vi "UpdateScrollbar.vi"(6 "# Cols":u32=1, 7 "Value Scrollbar":i32, 8 "error in":errorcluster, 9 "#Rows":u32=7, 10 "# Elements":i32, 11 "Cluster Refnum":refnum<vi>) -> (0 "error out":errorcluster)   [LabVIEW 2020, in "FakedArray.lvclass"]
uses:
  FakedArray.lvclass
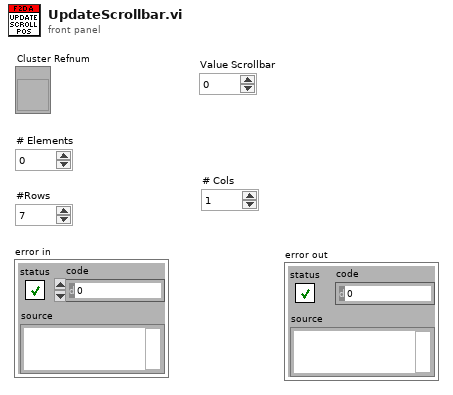
[diagram p1: front panel]
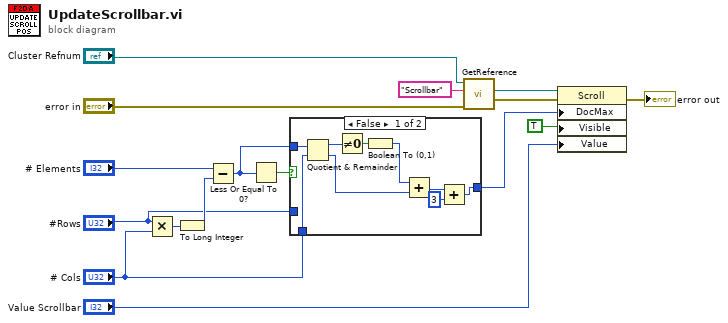
[diagram p0: block diagram]
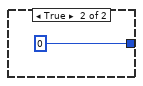
[diagram p2: hidden frame]
diagram:
  n1 = Multiply(x="#Rows", y="# Cols") -> (x*y=w2:u32)
  n2 = To Long Integer(number=w2) -> (32bit integer=w5:i32)
  n3 = Subtract(x="# Elements", y=w5) -> (x-y=w16:i32)
  n4 = Less Or Equal To 0?(x=w16) -> (x <= 0?=w13:bool)
  n5 = case shown="False" w13 {
    tunnel: [w18 0] -> w14
    tunnel: w16 -> [w25 _]
    tunnel: "# Cols" -> [w24 _]
    tunnel: "#Rows" -> [_ _]
    frame False {
      n6 = Quotient & Remainder(x=w25, y=w24) -> (x-y*floor(x/y)=w23:u32, floor(x/y)=w20:u32)
      n7 = Not Equal To 0?(x=w23) -> (x != 0?=w22:bool)
      n8 = Boolean To (0,1)(Boolean=w22) -> (0, 1=w21:i16)
      n9 = Add(x=w21, y=w20) -> (x+y=w19:u32)
      n10 = Add(x=w19, y=u32 3) -> (x+y=w18:u32)
    }
    frame True {
    }
  }
  n11 = call "GetReference.vi"("error in (no error)"="error in", "Label"="Scrollbar", "Framework Templates"="Cluster Refnum") -> ("error out"=w9:errorcluster, "Scrollbar"=w8:refnum<vi>)  [unwired: 7 out]
  n12 = property class="Scroll"(reference=w8, error in=w9, "DocMax"=w14, "Visible"=TRUE ("Coerce Maximum Value"), "Value"="Value Scrollbar") -> (error out=→"error out":errorcluster)  [unwired: 1 out]
